vi "Read Channel.vi"(8 "error in":errorcluster, 10 "Channel":variant, 11 "DI DAQmx Cont CFG in":refnum<class "DI DAQmx Cont CFG.lvclass">) -> (0 "error out":errorcluster, 2 "Reading":variant, 3 "DI DAQmx Cont CFG out":refnum<class "DI DAQmx Cont CFG.lvclass">)   [LabVIEW 2024, in "DI DAQmx Cont CFG.lvclass"]
uses:
  DI DAQmx Cont CFG.lvclass
  DI DAQmx Cont CFG.lvclass/DI DAQmx Cont CFG.ctl
  Buffers/Buffer Lossless Digital/Buffer Lossless Digital.lvclass
  DAQmx Base CFG/DAQmx Base CFG.lvclass
  <vilib>/DAQmx/read.llb/DAQmx Read (Digital 1D Wfm NChan NSamp).vi
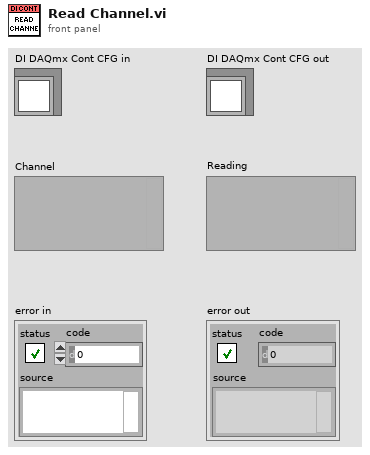
[diagram p1: front panel]
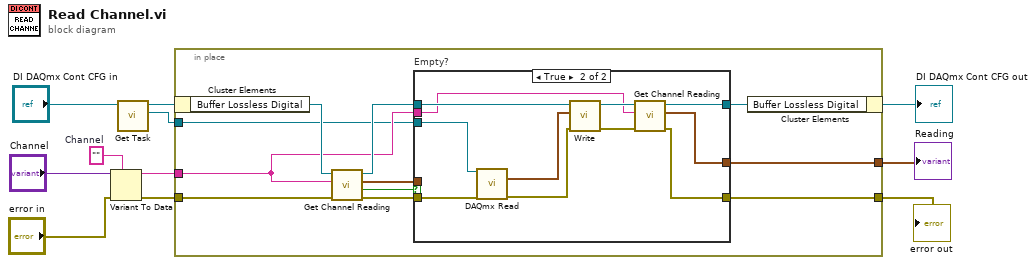
[diagram p0: block diagram]
diagram:
  w11 = ""  # Channel
  n1 = Variant To Data(error in="error in", type=w11, Variant="Channel") -> (data=w9:string, error out=w8:errorcluster)
  n2 = call "Get Task.vi"("DAQmx Base CFG in"="DI DAQmx Cont CFG in") -> ("Task"=w7:refnum<k21>, "DAQmx Base CFG out"=w10:refnum<class "DI DAQmx Cont CFG.lvclass">)  [unwired: 9 in]
  n3 = in-place {
    in-place-border: [w22] -> w2
    in-place-border: w9 -> [w16]
    in-place-border: [w19] -> w1
    in-place-border: w8 -> [w17]
    in-place-border: w7 -> [w14]
    n4 = in-place-cluster #1(w10) -> ("Buffer Lossless Digital"=w21:refnum<class "Buffer Lossless Digital.lvclass">)
    n5 = call "Get Channel Reading.vi"("error in"=w17, "Channel"=w16, "Buffer Lossless Bin in"=w21) -> ("error out"=w15:errorcluster, "empty?"=w13:bool, "Reading"=w12:digitalwaveform, "Buffer Lossless Bin out"=w18:refnum<class "Buffer Lossless Digital.lvclass">)  [unwired: 5 in]
    n6 = case "Empty?" shown="True" w13 {
      tunnel: [w23 w36] -> w22
      tunnel: [w24 w35] -> w20
      tunnel: [w25 w26] -> w19
      tunnel: w18 -> [w24 w30]
      tunnel: w16 -> [_ w27]
      tunnel: w15 -> [w23 w34]
      tunnel: w14 -> [_ w33]
      tunnel: w12 -> [w25 _]
      frame False {
      }
      frame True {
        n7 = call-poly <vilib>:"DAQmx Read.vi"("task/channels in"=w33, "error in"=w34) -> ("data"=w28:digitalwaveform[], "error out"=w32:errorcluster)  [unwired: 11 in, 1 out]
        n8 = call "Write.vi"("error in"=w32, "Readings"=w28, "Buffer Lossless Digital in"=w30) -> ("error out"=w31:errorcluster, "Buffer Lossless Digital out"=w29:refnum<class "Buffer Lossless Digital.lvclass">)  [unwired: 7 in]
        n9 = call "Get Channel Reading.vi"("error in"=w31, "Channel"=w27, "Buffer Lossless Bin in"=w29) -> ("error out"=w36:errorcluster, "Reading"=w26:digitalwaveform, "Buffer Lossless Bin out"=w35:refnum<class "Buffer Lossless Digital.lvclass">)  [unwired: 5 in, 1 out]
      }
    }
    n10 = in-place-cluster #1("Buffer Lossless Digital"=w20) -> (→"DI DAQmx Cont CFG out":refnum<class "DI DAQmx Cont CFG.lvclass">)
  }
  "error out" <- w2
  "Reading" <- w1
